vi "Search Coord.vi"(8 "error in (no error)":errorcluster, 11 "PNG Path":path) -> (0 "error out":errorcluster, 1 "PNG picture":picture, 2 "Puck 2":cluster{"X2":dbl, "Y2":dbl}, 3 "Puck 1":cluster{"X1":dbl, "Y1":dbl}, 5 "Warning (C++)":string)   [LabVIEW 2017]
panel:
  out "Executable name":string
  out "Actual executable path":path
  out "match substring":string
  out "VI name":string
  in  "color 2":u32=1
  in  "color 1":u32
  out "PNG path":path
  out "standard error":string
  out "standard output":string
  out "Pos":string
  out "hauteur":i16
  out "largeur":i16
  out "image":u8[](array[numeric])
  out "image depth":i32
  out "Pixmap":u32[](array[numeric])
  # "M. Zemp & I. Scholl GM BA 2"
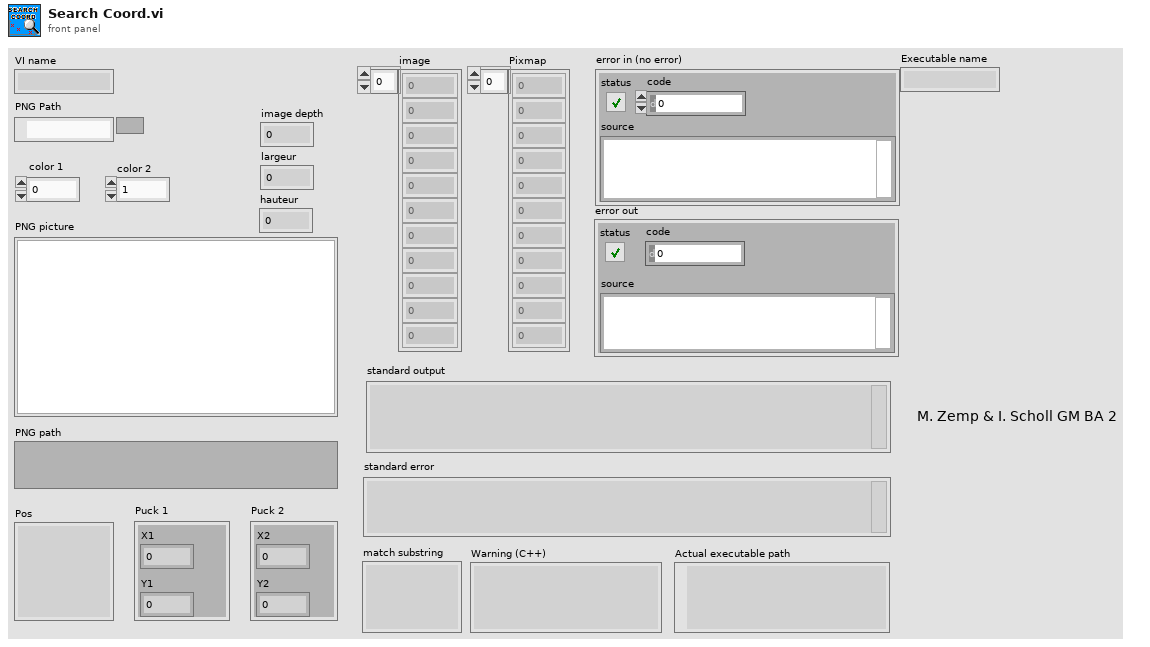
[diagram p1: front panel]
types:
  T1 = enum16{"big-endian, network order", "native, host order", "little-endian"}
  T2 = enum16{"open", "replace", "create", "open or create", "replace or create", "replace or create with confirmation"}
  T3 = typedef "imagedata.ctl" = cluster{"image type":i32, "image depth":i32, "image":u8[], "mask":u8[], "colors":u32[], "Rectangle":cluster{"left":i16, "top":i16, "right":i16, "bottom":i16}}
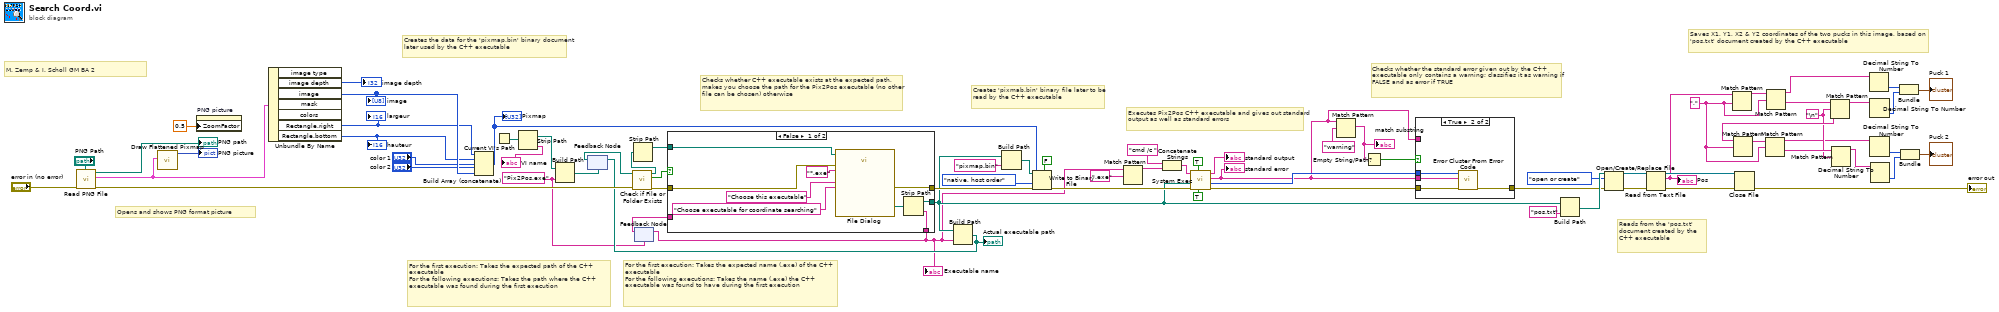
[diagram p0: block diagram]
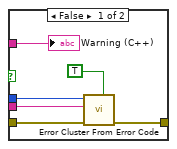
[diagram p2: hidden frame]
diagram:
  w3 = "Pix2Pos.exe"
  w54 = "\n"
  w59 = "," ("regular expression")
  # "M. Zemp & I. Scholl GM BA 2"
  # "Creates 'pixmab.bin' binary file later to be read by the C++ executable"
  # "Reads from the 'pos.txt' document created by the C++ executable"
  # "For the first execution: Takes the expected name (.exe) of the C++ executable\nFor the following executions: Takes the name (.exe) the C++ executable was found to have during the first execution"
  # "Saves X1, Y1, X2 & Y2 coordinates of the two pucks in this image, based on 'pos.txt' document created by the C++ executable"
  # "Checks whether the standard error given out by the C++ executable only contains a warning; classifies it as warning if FALSE and as error if TRUE"
  # "Executes Pix2Pos C++ executable and gives out standard output as well as standard errors"
  # "Checks whether C++ executable exists at the expected path, makes you choose the path for the Pix2Pos executable (no other file can be chosen) otherwise"
  # "For the first execution: Takes the expected path of the C++ executable\nFor the following executions: Takes the path where the C++ executable was found during the first execution"
  # "Creates the data for the 'pixmap.bin' binary document later used by the C++ executable"
  # "Opens and shows PNG format picture"
  n1 = call <vilib>:"Read PNG File.vi"("error in (no error)"="error in (no error)", "path to PNG file"="PNG Path") -> ("error out"=w65:errorcluster, "image data"=w72:T3, "path"=→"PNG path":path)  [unwired: 7 in]
  n2 = call <vilib>:"Draw Flattened Pixmap.vi"("image data"=w72) -> ("new picture"=→"PNG picture":picture)  [unwired: 8 in]
  n3 = property on="PNG picture" class="Pict"("ZoomFactor"=sgl 0.5 ("Zoom Factor")) -> ()  [unwired: 2 in, 2 out]
  n4 = Unbundle By Name(w72) -> ("image depth"=→"image depth":i32, "image"=w70:u8[], "Rectangle.right"=w69:i16, "Rectangle.bottom"=w68:i16)  [unwired: 3 out]
  "image" <- w70
  "largeur" <- w69
  "hauteur" <- w68
  n5 = Build Array (concatenate)(w69, w68, "color 1", "color 2", w70) -> (w11:u32[])
  "Pixmap" <- w11
  n6 = Current VI's Path() -> (path=w67:path)
  n7 = Strip Path(path=w67) -> (stripped path=w26:path, name=→"VI name":string)
  n8 = Build Path(base path=w26, name or relative path=w3) -> (appended path=w19:path)
  n9 = feedback #1(w19) -> (w18:path)
  n10 = call <vilib>:"Check if File or Folder Exists.vi"("error in (no error)"=w65, "path"=w18) -> ("error out"=w31:errorcluster, "file or folder exists?"=w32:bool, "dup path"=w16:path)  [unwired: 7 in]
  n11 = Strip Path(path=w16) -> (stripped path=w17:path)  [unwired: 1 out]
  n12 = feedback #2(w3) -> (w2:string)
  n13 = case shown="False" w32 {
    tunnel: w31 -> [w83 w86]
    tunnel: [w82 w86] -> w9
    tunnel: [w81 w85] -> w7
    tunnel: w17 -> [w80 w85]
    tunnel: [w77 w84] -> w1
    tunnel: w2 -> [_ w84]
    frame False {
      n14 = call "File Dialog"("start path"=w80, "prompt"="Choose executable for coordinate searching", "button label"="Choose this executable", "error in"=w83, "pattern (all files)"="*.exe") -> ("selected path"=w76:path, "error out"=w82:errorcluster)  [unwired: 7 in, 2 out]
      n15 = Strip Path(path=w76) -> (stripped path=w81:path, name=w77:string)
    }
    frame True {
    }
  }
  "Executable name" <- w1
  n16 = feedback-in #2(w1) -> ()
  n17 = Build Path(base path=w7, name or relative path=w1) -> (appended path=w15:path)
  "Actual executable path" <- w15
  n18 = feedback-in #1(w15) -> ()
  n19 = Build Path(base path=w7, name or relative path="pixmap.bin") -> (appended path=w12:path)
  n20 = Write to Binary File(file (use dialog)=w12, data=w11, error in=w9, 5:FALSE ("prepend array or string size? (T)"), 9:T1."native, host order" ("byte order (0:big-endian, network order)")) -> (error out=w8:errorcluster)  [unwired: 1 in, 2 out]
  n21 = Match Pattern(string=w1, regular expression=".exe") -> (before substring=w5:string)  [unwired: 1 in, 3 out]
  n22 = Concatenate Strings("cmd /c " ("command line"), w5) -> (w6:string)
  n23 = call <vilib>:"System Exec.vi"("run minimized? (F)"=TRUE, "wait until completion? (T)"=TRUE, "error in (no error)"=w8, "working directory"=w7, "command line"=w6) -> ("error out"=w28:errorcluster, "return code"=w24:i32, "standard error"=w20:string, "standard output"=→"standard output":string)  [unwired: 3 in]
  "standard error" <- w20
  n24 = Match Pattern(string=w20, regular expression="warning") -> (match substring=w22:string)  [unwired: 1 in, 3 out]
  "match substring" <- w22
  n25 = Empty String/Path?(string/path=w22) -> (empty?=w21:bool)
  n26 = case shown="True" w21 {
    tunnel: w28 -> [w91 w96]
    tunnel: [w92 w95] -> w25
    tunnel: w20 -> [w90 w94]
    tunnel: w24 -> [w89 w93]
    tunnel: w20 -> [w87 _]
    frame False {
      n27 = call <vilib>:"Error Cluster From Error Code.vi"("is warning? (False)"=TRUE, "error in (no error)"=w91, "error message (\"\")"=w90, "error code (0)"=w89) -> ("error out"=w92:errorcluster)  [unwired: 5 in]
      "Warning (C++)" <- w87
    }
    frame True {
      n28 = call <vilib>:"Error Cluster From Error Code.vi"("error in (no error)"=w96, "error message (\"\")"=w94, "error code (0)"=w93) -> ("error out"=w95:errorcluster)  [unwired: 6 in]
    }
  }
  n29 = Build Path(base path=w7, name or relative path="pos.txt") -> (appended path=w43:path)
  n30 = Open/Create/Replace File(file path (use dialog)=w43, error in=w25, operation (0:open)=T2."open or create") -> (refnum out=w42:refnum<file>, error out=w36:errorcluster)  [unwired: 3 in, 1 out]
  n31 = Read from Text File(file (use dialog)=w42, error in=w36) -> (refnum out=w41:refnum<file>, text=w40:string, error out=w39:errorcluster)  [unwired: 2 in, 1 out]
  "Pos" <- w40
  n32 = Match Pattern(string=w40, regular expression=w59) -> (after substring=w63:string)  [unwired: 1 in, 3 out]
  n33 = Close File(refnum=w41, error in=w39) -> (error out=→"error out":errorcluster)  [unwired: 1 out]
  n34 = Match Pattern(string=w63, regular expression=w59) -> (before substring=w53:string, after substring=w62:string)  [unwired: 1 in, 2 out]
  n35 = Match Pattern(string=w62, regular expression=w54) -> (before substring=w50:string, after substring=w61:string)  [unwired: 1 in, 2 out]
  n36 = Match Pattern(string=w61, regular expression=w59) -> (after substring=w60:string)  [unwired: 1 in, 3 out]
  n37 = Match Pattern(string=w60, regular expression=w59) -> (before substring=w48:string, after substring=w58:string)  [unwired: 1 in, 2 out]
  n38 = Match Pattern(string=w58, regular expression=w54) -> (before substring=w47:string)  [unwired: 1 in, 3 out]
  n39 = Decimal String To Number(string=w53) -> (number=w51:i32)  [unwired: 2 in, 1 out]
  n40 = Decimal String To Number(string=w50) -> (number=w49:i32)  [unwired: 2 in, 1 out]
  n41 = Decimal String To Number(string=w48) -> (number=w46:i32)  [unwired: 2 in, 1 out]
  n42 = Decimal String To Number(string=w47) -> (number=w45:i32)  [unwired: 2 in, 1 out]
  n43 = Bundle(w51, w49) -> (→"Puck 1":cluster{i32, i32})  [unwired: 1 in]
  n44 = Bundle(w46, w45) -> (→"Puck 2":cluster{i32, i32})  [unwired: 1 in]
